vi "WillDey_IV_Curve.vi"() -> ()   [LabVIEW 2017]
panel:
  out "Measured Voltage":dbl format="%#_g V"
  out "Goal Voltage":dbl format="%#_g V"
  in  "Reverse":bool
  in  "Stop":bool
  out "I-V Curve":cluster{"X":dbl, "Y":dbl}[](graph)
  in  "Delay Time (s)":dbl=0.001
  in  "Step":dbl
  in  "Final Voltage":dbl
  in  "Instrument":refnum<k15>="\"GPIB::14::INSTR\"" caption="resource name (\"GPIB::14::INSTR\")"
  in  "Start Voltage":dbl
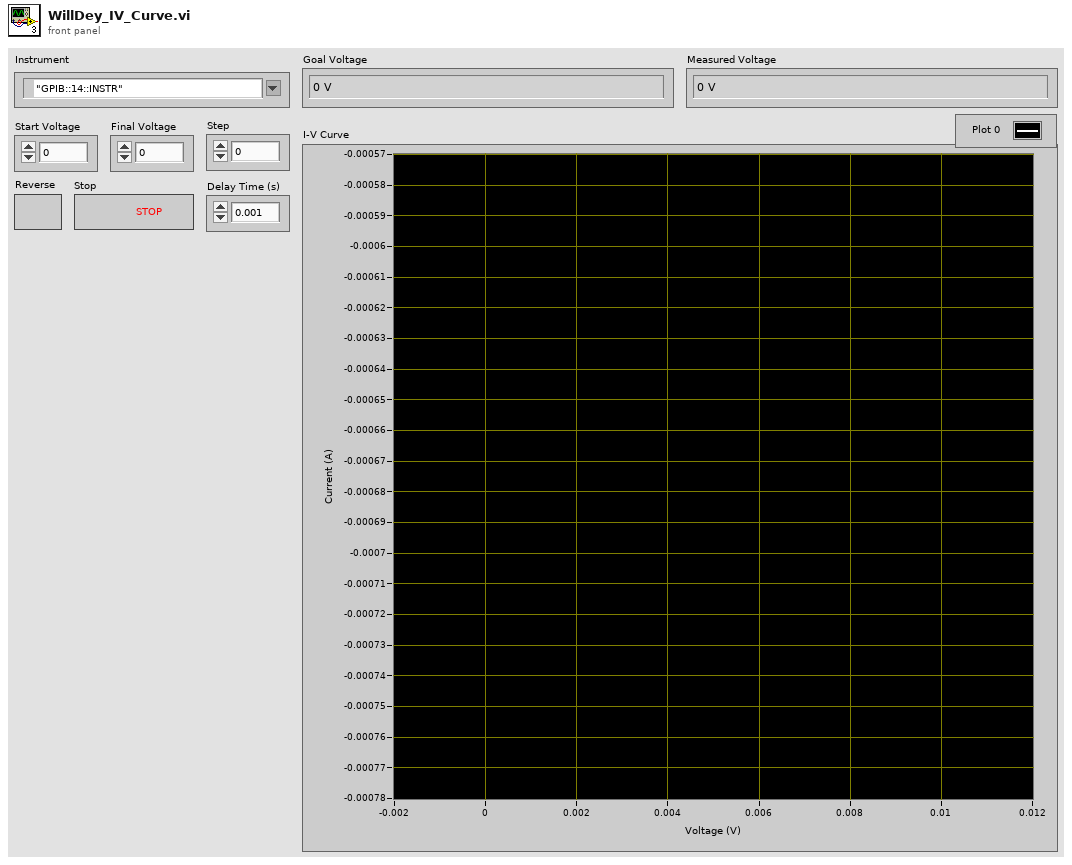
[diagram p1: front panel]
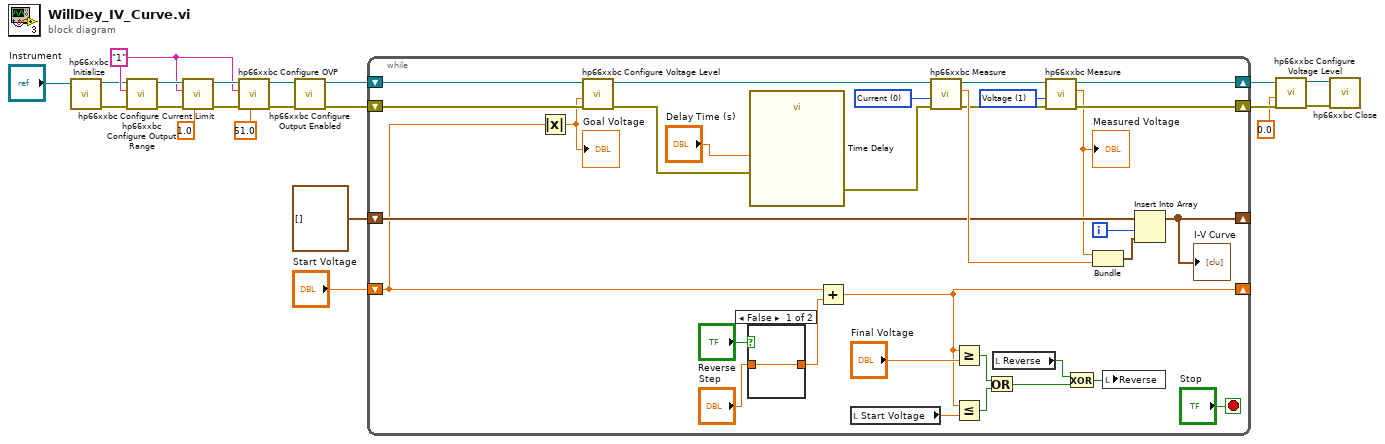
[diagram p0: block diagram]
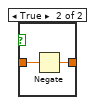
[diagram p2: hidden frame]
diagram:
  w15 = "1" ("channel (\"\") name")
  n1 = call <instrlib>:"hp66xxbc Initialize.vi"("resource name (\"GPIB::14::INSTR\")"="Instrument") -> ("error out"=w13:errorcluster, "instrument handle"=w12:refnum<k15>)  [unwired: 9 in]
  n2 = call <instrlib>:"hp66xxbc Configure Output Range.vi"("error in (no error)"=w13, "channel name (\"\")"=w15, "instrument handle"=w12) -> ("error out"=w17:errorcluster, "instrument handle out"=w18:refnum<k15>)  [unwired: 7 in]
  n3 = call <instrlib>:"hp66xxbc Configure Current Limit.vi"("limit (0.00 A)"=1.0, "error in (no error)"=w17, "channel name (\"\")"=w15, "instrument handle"=w18) -> ("error out"=w19:errorcluster, "instrument handle out"=w20:refnum<k15>)  [unwired: 6 in]
  n4 = call <instrlib>:"hp66xxbc Configure OVP.vi"("limit (0.0 V)"=51.0, "error in (no error)"=w19, "channel name (\"\")"=w15, "instrument handle"=w20) -> ("error out"=w10:errorcluster, "instrument handle out"=w11:refnum<k15>)  [unwired: 6 in]
  n5 = call <instrlib>:"hp66xxbc Configure Output Enabled.vi"("error in (no error)"=w10, "instrument handle"=w11) -> ("error out"=w8:errorcluster, "instrument handle out"=w9:refnum<k15>)  [unwired: 8 in]
  n6 = while {
    shift-right: [w38] -> w5
    shift-left: w8 -> [w53]
    shift-right: [w39] -> w6
    shift-left: w9 -> [w52]
    shift-right: [w42] -> _
    shift-left: cluster{dbl, "measurement":dbl}[] [] ("array") -> [w43]
    shift-right: [w29] -> _
    shift-left: "Start Voltage" -> [w22]
    i -> [w46]
    stop <- "Stop" stop-if-true
    w37 = 1 items=["Voltage"=1, "Current"=0] ("measurement type (1:voltage)")
    w50 = 0 items=["Voltage"=1, "Current"=0] ("measurement type (1:voltage)")
    n7 = Absolute Value(x=w22) -> (abs(x)=w28:dbl)
    "Goal Voltage" <- w28
    n8 = call <instrlib>:"hp66xxbc Configure Voltage Level.vi"("error in (no error)"=w53, "level (0.0)"=w28, "instrument handle"=w52) -> ("error out"=w48:errorcluster, "instrument handle out"=w51:refnum<k15>)  [unwired: 7 in]
    n9 = case shown="False" "Reverse" {
      tunnel: "Step" -> [w54 w56]
      tunnel: [w54 w55] -> w34
      frame False {
      }
      frame True {
        n10 = Negate(x=w56) -> (-x=w55:dbl)
      }
    }
    n11 = call "Time Delay"("error in (no error)"=w48, "Delay Time (s)"="Delay Time (s)") -> ("error out"=w47:errorcluster)  [unwired: 9 in]
    n12 = Add(x=w22, y=w34) -> (x+y=w29:dbl)
    n13 = local read "Start Voltage"() -> (w32:dbl)
    n14 = call <instrlib>:"hp66xxbc Measure.vi"("error in (no error)"=w47, "measurement type (1:voltage)"=w50, "instrument handle"=w51) -> ("error out"=w40:errorcluster, "measurement"=w45:dbl, "instrument handle out"=w41:refnum<k15>)  [unwired: 6 in]
    n15 = Greater Or Equal?(x=w29, y="Final Voltage") -> (x >= y?=w30:bool)
    n16 = Less Or Equal?(x=w29, y=w32) -> (x <= y?=w31:bool)
    n17 = Or(x=w30, y=w31) -> (x .or. y?=w26:bool)
    n18 = local read "Reverse"() -> (w24:bool)
    n19 = call <instrlib>:"hp66xxbc Measure.vi"("error in (no error)"=w40, "measurement type (1:voltage)"=w37, "instrument handle"=w41) -> ("error out"=w38:errorcluster, "measurement"=w23:dbl, "instrument handle out"=w39:refnum<k15>)  [unwired: 6 in]
    "Measured Voltage" <- w23
    n20 = Exclusive Or(1:w26, 2:w24) -> (0:w25:bool)
    n21 = Bundle("measurement"=w23, "measurement"=w45) -> (w44:cluster{"measurement":dbl, "measurement":dbl})  [unwired: 1 in]
    n22 = local write "Reverse"(w25) -> ()
    n23 = Insert Into Array(array=w43, index=w46, new element=w44) -> (w42:cluster{dbl, "measurement":dbl}[])
    "I-V Curve" <- w42
  }
  n24 = call <instrlib>:"hp66xxbc Configure Voltage Level.vi"("error in (no error)"=w5, "level (0.0)"=0.0, "instrument handle"=w6) -> ("error out"=w3:errorcluster, "instrument handle out"=w4:refnum<k15>)  [unwired: 7 in]
  n25 = call <instrlib>:"hp66xxbc Close.vi"("error in (no error)"=w3, "instrument handle"=w4) -> ()  [unwired: 9 in, 1 out]
